vi "CRC_Calculation.vi"(11 "CMD":string="\u0000") -> (3 "CMD + CRC":string)   [LabVIEW 2021]
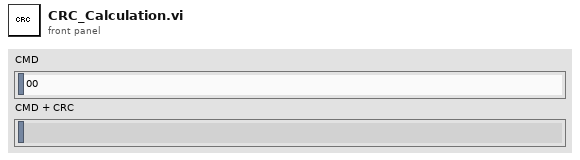
[diagram p1: front panel]
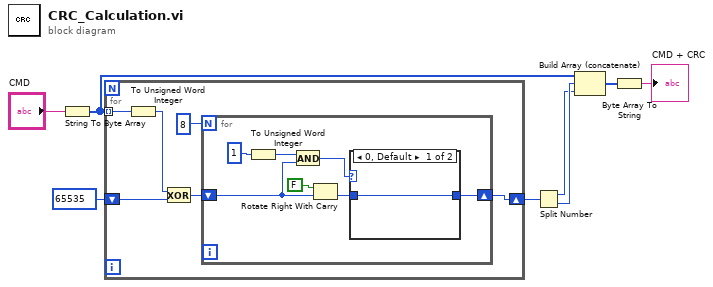
[diagram p0: block diagram]
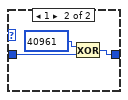
[diagram p2: hidden frame]
diagram:
  n1 = String To Byte Array(string="CMD") -> (unsigned byte array=w3:u8[])
  n2 = for {
    shift-right: [w13] -> w8
    shift-left: u16 65535 -> [w11]
    tunnel: w3 -> [w10] mode=indexing
    n3 = To Unsigned Word Integer(number=w10) -> (unsigned 16bit integer=w9:u16)
    n4 = Exclusive Or(1:w11, 2:w9) -> (0:w12:u16)
    n5 = for {
      N: 8 -> [_]
      shift-right: [w20] -> w13
      shift-left: w12 -> [w19]
      n6 = To Unsigned Word Integer(number=1) -> (unsigned 16bit integer=w16:u16)
      n7 = And(x=w16, y=w19) -> (x .and. y?=w18:u16)
      n8 = Rotate Right With Carry(2:w19, 3:FALSE ("Übertrag")) -> (0:w21:u16)  [unwired: 1 out]
      n9 = case shown="0, Default" w18 {
        tunnel: w21 -> [w22 w24]
        tunnel: [w22 w25] -> w20
        frame 0, Default {
        }
        frame 1 {
          n10 = Exclusive Or(1:w24, 2:u16 40961) -> (0:w25:u16)
        }
      }
    }
  }
  n11 = Split Number(x=w8) -> (hi(x)=w5:u8, lo(x)=w6:u8)
  n12 = Build Array (concatenate)(w3, w6, w5) -> (w4:u8[])
  n13 = Byte Array To String(unsigned byte array=w4) -> (string=→"CMD + CRC":string)
